vi "Get TX Message.vi"(8 "error in (no error)":errorcluster, 11 "RxTx in":refnum<class "RxTx.lvclass">) -> (0 "error out":errorcluster, 3 "RxTx out":refnum<class "RxTx.lvclass">)   [LabVIEW 2018, in "RxTx.lvclass"]
doc: "Pop the lastest Tx message found in the qeue"
uses:
  RxTx.lvclass
  RxTx.lvclass/RxTx.ctl
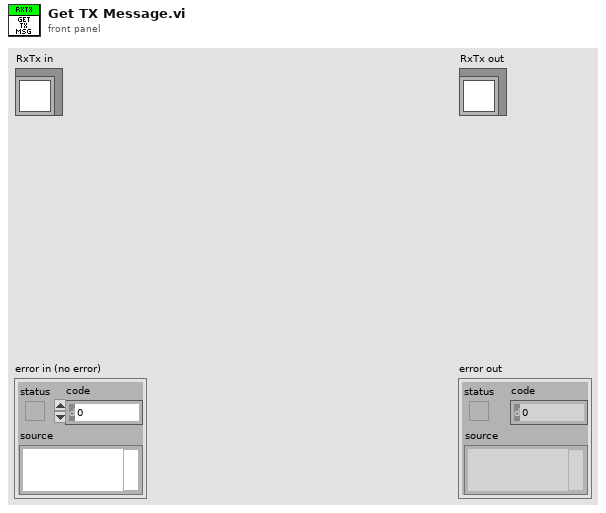
[diagram p1: front panel]
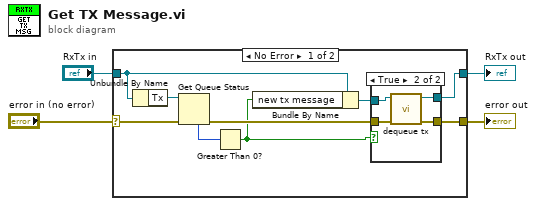
[diagram p0: block diagram]
diagram:
  n1 = case shown="No Error" "error in (no error)" {
    selector: "error in (no error)" -> [w11 w21]
    tunnel: [w9 w21] -> w2
    tunnel: [w13 w20] -> w1
    tunnel: "RxTx in" -> [w8 w20]
    frame No Error {
      n2 = Unbundle By Name(w8) -> ("Tx"=w12:refnum<queue>)
      n3 = Get Queue Status(queue=w12, error in (no error)=w11) -> (error out=w10:errorcluster, # elements in queue=w6:i32)  [unwired: 1 in, 6 out]
      n4 = Greater Than 0?(x=w6) -> (x > 0?=w5:bool)
      n5 = Bundle By Name(cluster=w8, "new tx message"=w5) -> (w7:refnum<class "RxTx.lvclass">)
      n6 = case shown="True" w5 {
        tunnel: w7 -> [w14 w19]
        tunnel: [w14 w16] -> w13
        tunnel: w10 -> [w15 w18]
        tunnel: [w15 w17] -> w9
        frame False {
        }
        frame True {
          n7 = call "dequeue tx.vi"("error in (no error)"=w18, "RxTx in"=w19) -> ("error out"=w17:errorcluster, "RxTx out"=w16:refnum<class "RxTx.lvclass">)  [unwired: 8 in]
        }
      }
    }
    frame Error {
    }
  }
  "error out" <- w2
  "RxTx out" <- w1
